vi "switchLED.vi"(8 "error in (no error)":errorcluster, 10 "Which LED":u8, 11 "Arduino session":refnum<visa-resource-name>) -> (0 "error out":errorcluster, 2 "LED vector":bool[](array[boolean]), 3 "Arduino session":refnum<visa-resource-name>)   [LabVIEW 2017]
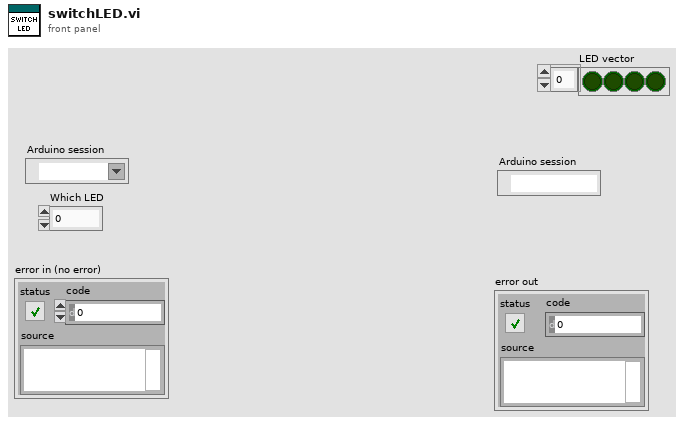
[diagram p1: front panel]
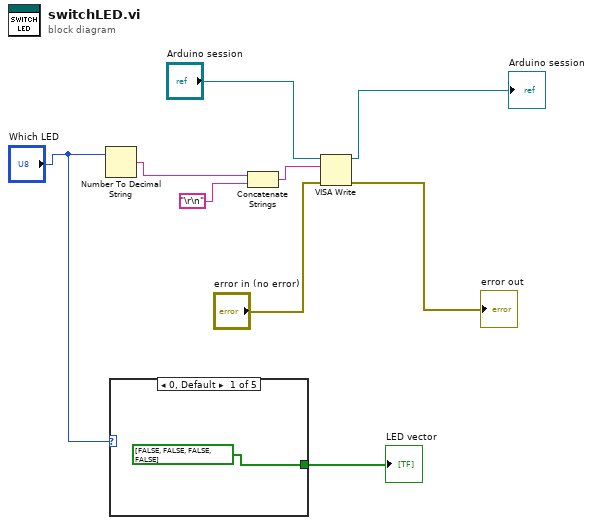
[diagram p0: block diagram]
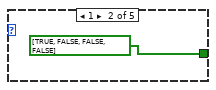
[diagram p2: hidden frame]
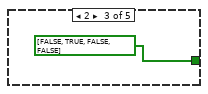
[diagram p3: hidden frame]
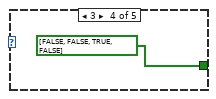
[diagram p4: hidden frame]
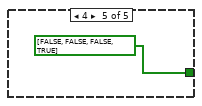
[diagram p5: hidden frame]
diagram:
  n1 = Number To Decimal String(number="Which LED") -> (decimal integer string=w3:string)  [unwired: 1 in]
  n2 = case shown="0, Default" "Which LED" {
    tunnel: [bool[] [FALSE, FALSE, FALSE, FALSE] bool[] [TRUE, FALSE, FALSE, FALSE] bool[] [FALSE, TRUE, FALSE, FALSE] bool[] [FALSE, FALSE, TRUE, FALSE] bool[] [FALSE, FALSE, FALSE, TRUE]] -> w1
    frame 0, Default {
    }
    frame 1 {
    }
    frame 2 {
    }
    frame 3 {
    }
    frame 4 {
    }
  }
  "LED vector" <- w1
  n3 = Concatenate Strings(w3, "\r\n") -> (w8:string)
  n4 = VISA Write(VISA resource name="Arduino session", write buffer=w8, error in (no error)="error in (no error)") -> (VISA resource name out=→"Arduino session":refnum<visa-resource-name>, error out=→"error out":errorcluster)  [unwired: 1 out]
